vi "Handle Server Request.vi"(7 "parameters":string[][](array[string]), 8 "error in (no error)":errorcluster, 10 "id in":i32, 11 "request":string) -> (0 "error out":errorcluster, 3 "response":string)   [LabVIEW 2025, in "MCP Server.lvlib"]
doc: "Use this VI to handle an MCP RPC message. This VI accepts a json with request data and replies with a json object with response data. It implements the full MCP server. Use the MCP server api in your code to register tools and prompts and make them available in the server."
uses:
  MCP Server.lvlib
  17ff933e-622e-44bb-904e-4e6adce09461.vi
  <vilib>/JDP Science/JSONtext/Next JSON Value.vi
  <vilib>/JDP Science/JSONtext/String Subset.vi
  <vilib>/JDP Science/JSONtext/Parsing/Advance past next JSON Value (inlined COPY).vi
  <vilib>/JDP Science/JSONtext/Parsing/Advance past whitespace.vi
  <vilib>/JDP Science/JSONtext/Parsing/Advance past String.vi
  <vilib>/JDP Science/JSONtext/Parsing/Advance past Number.vi
  <vilib>/JDP Science/JSONtext/Parsing/Advance past Line Ending.vi
  <vilib>/JDP Science/JSONtext/Parsing/Parse Full Path or Item Name.vi
  <vilib>/JDP Science/JSONtext/Parsing/Advance past Array.vi
  <vilib>/JDP Science/JSONtext/Parsing/Advance past Object.vi
  <vilib>/JDP Science/JSONtext/support/Error Cluster From Code.vi
  <vilib>/JDP Science/JSONtext/Offset/Find Item Locations by Path.vi
  <vilib>/JDP Science/JSONtext/JSON text to Variant.vi
  <vilib>/JDP Science/JSONtext/LVClass Serializer/JSONtext LVClass Serializer.lvclass
  <vilib>/JDP Science/JSONtext/JSONtext.lvlib
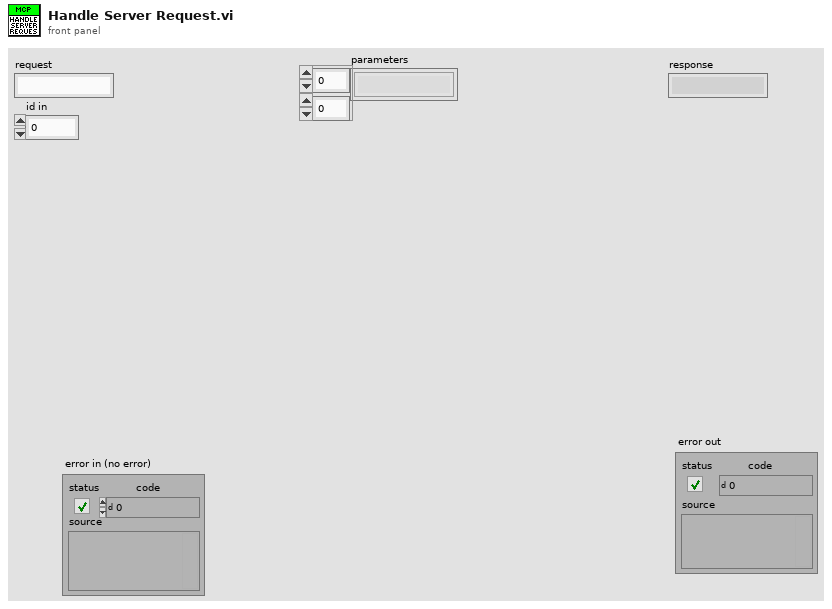
[diagram p1: front panel]
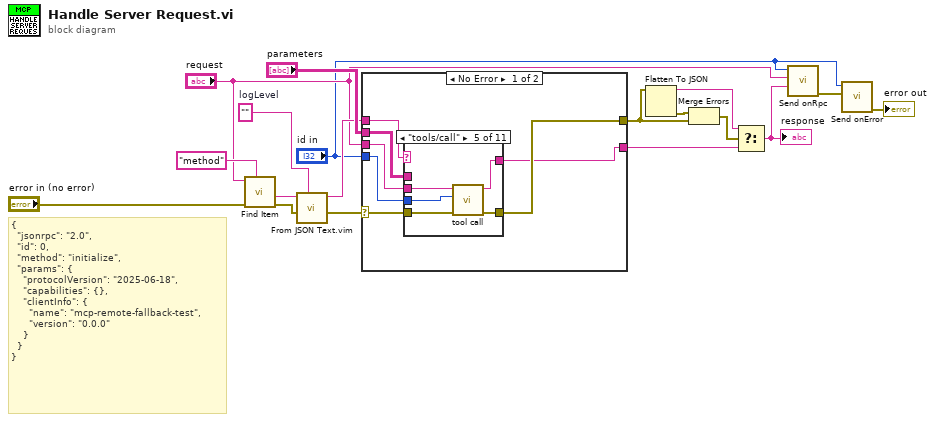
[diagram p0: block diagram]
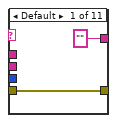
[diagram p2: hidden frame]
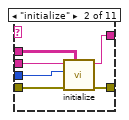
[diagram p3: hidden frame]
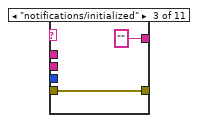
[diagram p4: hidden frame]
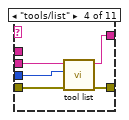
[diagram p5: hidden frame]
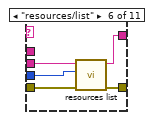
[diagram p6: hidden frame]
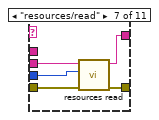
[diagram p7: hidden frame]
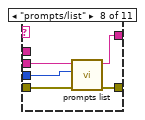
[diagram p8: hidden frame]
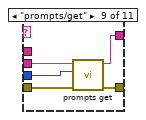
[diagram p9: hidden frame]
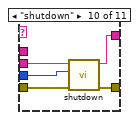
[diagram p10: hidden frame]
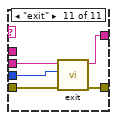
[diagram p11: hidden frame]
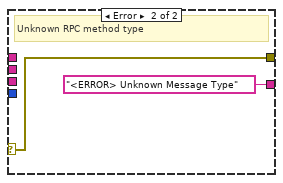
[diagram p12: hidden frame]
diagram:
  w12 = ""  # logLevel
  # "{\n  \"jsonrpc\": \"2.0\",\n  \"id\": 0,\n  \"method\": \"initialize\",\n  \"params\": {\n    \"protocolVersion\": \"2025-06-18\",\n    \"capabilities\": {},\n    \"clientInfo\": {\n      \"name\": \"mcp-remote-fallback-test\",\n      \"version\": \"0.0.0\"\n    }\n  }\n}"
  n1 = call <vilib>:"Find Item.vi"("$Path or Item Name"="method", "error in (no error)"="error in (no error)", "JSON"="request") -> ("error out"=w11:errorcluster, "<JSON>"=w13:string)  [unwired: 5 in, 2 out]
  n2 = call "From JSON Text.vim"("Data Type and Default Value"=w12, "error in (no error)"=w11, "JSON"=w13) -> ("error out"=w15:errorcluster, "Data out"=w16:string)  [unwired: 7 in]
  n3 = case shown="No Error" w15 {
    selector: w15 -> [w24 w77]
    tunnel: "request" -> [w25 _]
    tunnel: [w23 w77] -> w3
    tunnel: [w22 "<ERROR> Unknown Message Type" ("response")] -> w8
    tunnel: "id in" -> [w21 _]
    tunnel: w16 -> [w20 _]
    tunnel: "parameters" -> [w19 _]
    frame No Error {
      n4 = case shown="\"tools/call\"" w20 {
        tunnel: w25 -> [_ w33 _ w40 w45 w50 w55 w60 w64 w70 w75]
        tunnel: ["" ("response") w32 "" ("response") w37 w42 w48 w53 w59 w62 w67 w72] -> w22
        tunnel: w24 -> [w27 w31 w35 w39 w44 w49 w54 w57 w65 w69 w74]
        tunnel: [w27 w30 w35 w38 w43 w47 w52 w58 w63 w68 w73] -> w23
        tunnel: w21 -> [_ w29 _ w36 w41 w46 w51 w56 w61 w66 w71]
        tunnel: w19 -> [_ w28 _ _ _ _ _ _ _ _ _]
        frame Default {
        }
        frame "initialize" {
          n5 = call "initialize.vi"("parameters"=w28, "error in"=w31, "server id"=w29, "message json"=w33) -> ("error out"=w30:errorcluster, "response"=w32:string)  [unwired: 6 in]
        }
        frame "notifications/initialized" {
        }
        frame "tools/list" {
          n6 = call "tool list.vi"("error in"=w39, "server id in"=w36, "message json"=w40) -> ("error out"=w38:errorcluster, "response"=w37:string)  [unwired: 7 in]
        }
        frame "tools/call" {
          n7 = call "tool call.vi"("error in"=w44, "id in"=w41, "message json"=w45) -> ("error out"=w43:errorcluster, "response"=w42:string)  [unwired: 7 in]
        }
        frame "resources/list" {
          n8 = call "resources list.vi"("error in"=w49, "server id"=w46, "message json"=w50) -> ("error out"=w47:errorcluster, "response"=w48:string)  [unwired: 7 in]
        }
        frame "resources/read" {
          n9 = call "resources read.vi"("error in"=w54, "id"=w51, "message json"=w55) -> ("error out"=w52:errorcluster, "response"=w53:string)  [unwired: 7 in]
        }
        frame "prompts/list" {
          n10 = call "prompts list.vi"("error in"=w57, "id"=w56, "message json"=w60) -> ("error out"=w58:errorcluster, "response"=w59:string)  [unwired: 7 in]
        }
        frame "prompts/get" {
          n11 = call "prompts get.vi"("error in"=w65, "id"=w61, "message json"=w64) -> ("error out"=w63:errorcluster, "response"=w62:string)  [unwired: 7 in]
        }
        frame "shutdown" {
          n12 = call "shutdown.vi"("error in"=w69, "id"=w66, "message json"=w70) -> ("error out"=w68:errorcluster, "response"=w67:string)  [unwired: 7 in]
        }
        frame "exit" {
          n13 = call "exit.vi"("error in"=w74, "id"=w71, "message json"=w75) -> ("error out"=w73:errorcluster, "response"=w72:string)  [unwired: 7 in]
        }
      }
    }
    frame Error {
      # "Unknown RPC method type"
    }
  }
  n14 = Flatten To JSON(anything=w3) -> (JSON string=w4:string, 11:w1:errorcluster)  [unwired: 2 in]
  n15 = Merge Errors(w1, w3) -> (w2:errorcluster)
  n16 = Select(t=w4, s=w2, f=w8) -> (s? t:f=w5:string)
  "response" <- w5
  n17 = call "Send onRpc.vi"("response"=w5, "request"="request", "id"="id in") -> ("error out"=w10:errorcluster)  [unwired: 8 in]
  n18 = call "Send onError.vi"("error to report"=w10, "id"="id in") -> ("error out"=→"error out":errorcluster)  [unwired: 9 in]
